vi "Report to the Control uService.vi"(8 "error in (no error)":errorcluster, 9 "Current Action":string, 10 "Monkey Status":T1=enum."Ongoing", 11 "Monkey in":refnum<class "Monkey.lvclass">=refnum) -> (0 "error out":errorcluster, 3 "Monkey out":refnum<class "Monkey.lvclass">)   [LabVIEW 2020, in "CIRCUS_uServices.lvlib" / "Monkey.lvlib" / "Monkey.lvclass"]
uses:
  Monkey.lvclass
  TALOS/TALOS_PPL.lvlibp/Father of all uServices/Father of all uServices/Father of all uServices.lvclass
  TALOS/TALOS_PPL.lvlibp
  TALOS/TALOS_PPL.lvlibp/Support VIs/Global Constants.vi
  C:/Users/marco/Documents/GitHub_Lab/CIRCUS/TALOS/TALOS_PPL.lvlibp/Father of all uServices/Father of all uServices/Father of all uServices.lvclass
  C:/Users/marco/Documents/GitHub_Lab/CIRCUS/TALOS/TALOS_PPL.lvlibp/Ancestor/Ancestor/Ancestor.lvclass
  C:/Users/marco/Documents/GitHub_Lab/CIRCUS/TALOS/Actor Framework.lvlibp/1abvi3w/vi.lib/ActorFramework/Actor/Actor.lvclass
  Run Utilities/Schedule/Schedule.lvclass
  Run Utilities/TypeDefs/Monkey Status.ctl
  Run Utilities/Run Utilities.lvlib
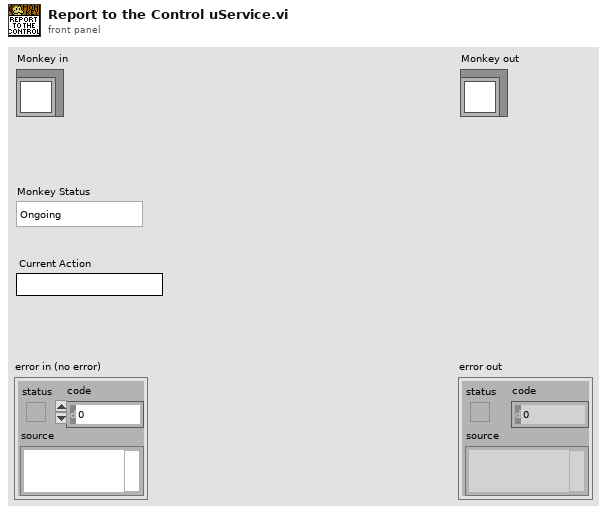
[diagram p1: front panel]
types:
  T1 = typedef "CIRCUS_uServices.lvlib/Run Utilities.lvlib/Monkey Status.ctl" = enum16{"Init", "Paused", "Ongoing", "Stopped", "Finished (no errors)", "Finished (with errors)"}
  T2 = typedef "CIRCUS_uServices.lvlib/Run Utilities.lvlib/Monkey Status Message.ctl" = cluster{"Monkey ID":string, "Monkey Status":T1, "Scripts left":u32, "ETA":string, "Current Action":string, "Report from previous RUNs":string, "Skipped RUNs":refnum<class "Schedule.lvclass">}
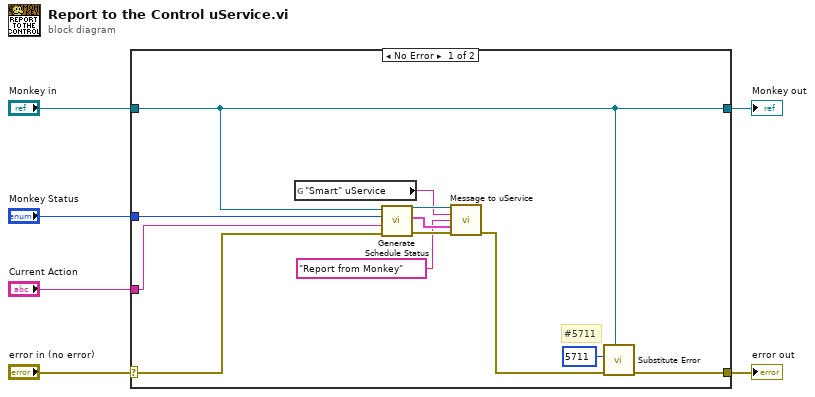
[diagram p0: block diagram]
diagram:
  n1 = case shown="No Error" "error in (no error)" {
    selector: "error in (no error)" -> [w14 w20]
    tunnel: [w13 w20] -> w5
    tunnel: [w11 w19] -> w3
    tunnel: "Monkey in" -> [w11 w19]
    tunnel: "Monkey Status" -> [w15 _]
    tunnel: "Current Action" -> [w8 _]
    frame No Error {
      # "#5711"
      n2 = global read "Global Constants.vi" "\"Smart\" uService"() -> (w7:string)
      n3 = call "Generate Schedule Status.vi"("error in (no error)"=w14, "Current Action"=w8, "Monkey Status"=w15, "Monkey in"=w11) -> ("error out"=w16:errorcluster, "Monkey Status Message"=w17:T2, "Monkey out"=w18:refnum<class "Monkey.lvclass">)  [unwired: 5 in]
      n4 = call "Message to uService.vi"("Father of all uServices in"=w18, "uService ID"=w7, "Message"="Report from Monkey", "Data"=w17, "error in (no error)"=w16) -> ("error out"=w12:errorcluster)  [unwired: 9 in, 1 out]
      n5 = call "Substitute Error.vi"("LabVIEW Object"=w11, "error in (no error)"=w12, "Error Code"=5711) -> ("error out"=w13:errorcluster)  [unwired: 8 in]
    }
    frame Error {
    }
  }
  "error out" <- w5
  "Monkey out" <- w3
